vi "equipotential.vi"(7 "Velocity":dbl, 10 "Pelletron Volts":dbl, 11 "Needle Voltes":dbl) -> (3 "Equipotential":dbl)   [LabVIEW 2011]
panel:
  # "2) \nEquipotential=4*pi*(2*8.85418782e-12*needlevolts*pelletronvolts./v.^2).^(3/2)*(3/7874)^(1/2);"
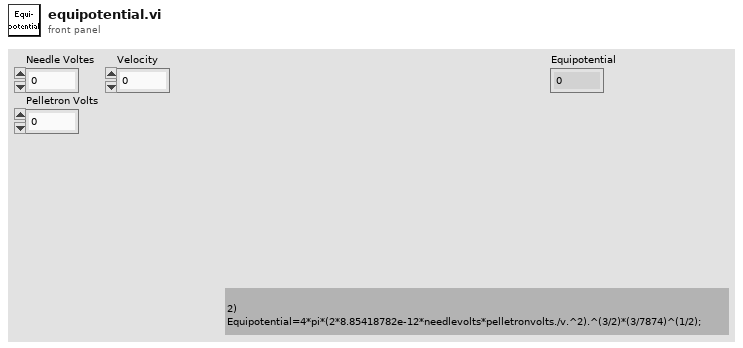
[diagram p1: front panel]
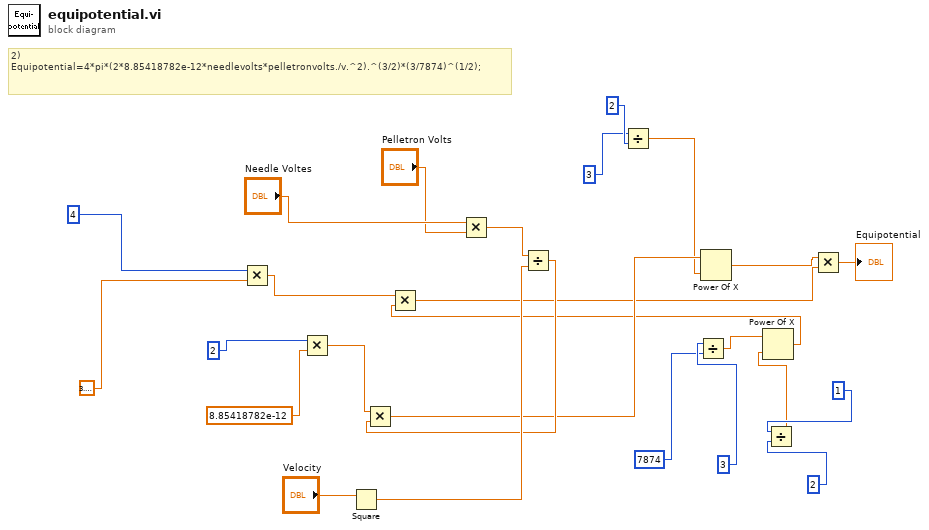
[diagram p0: block diagram]
diagram:
  # "2) \nEquipotential=4*pi*(2*8.85418782e-12*needlevolts*pelletronvolts./v.^2).^(3/2)*(3/7874)^(1/2);"
  n1 = Multiply(x=4, y=3.141592653589793) -> (x*y=w24:dbl)
  n2 = Multiply(x=2, y=8.85418782e-12) -> (x*y=w21:dbl)
  n3 = Square(x="Velocity") -> (x^2=w17:dbl)
  n4 = Multiply(x="Needle Voltes", y="Pelletron Volts") -> (x*y=w16:dbl)
  n5 = Divide(x=w16, y=w17) -> (x/y=w15:dbl)
  n6 = Multiply(x=w21, y=w15) -> (x*y=w14:dbl)
  n7 = Divide(x=3, y=2) -> (x/y=w11:dbl)
  n8 = Divide(x=3, y=7874) -> (x/y=w7:dbl)
  n9 = Power Of X(1:w11, 2:w14) -> (0:w10:dbl)
  n10 = Divide(x=1, y=2) -> (x/y=w4:dbl)
  n11 = Power Of X(1:w4, 2:w7) -> (0:w2:dbl)
  n12 = Multiply(x=w24, y=w2) -> (x*y=w1:dbl)
  n13 = Multiply(x=w10, y=w1) -> (x*y=→"Equipotential":dbl)
